vi "Move to Previous Positions.vi"(8 "error in (no error)":errorcluster) -> (0 "error out":errorcluster, 3 "Position Array":dbl[](array[numeric]))   [LabVIEW 2019, in "ESP301.lvlib"]
uses:
  ESP301.lvlib
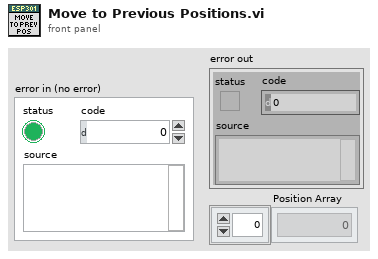
[diagram p1: front panel]
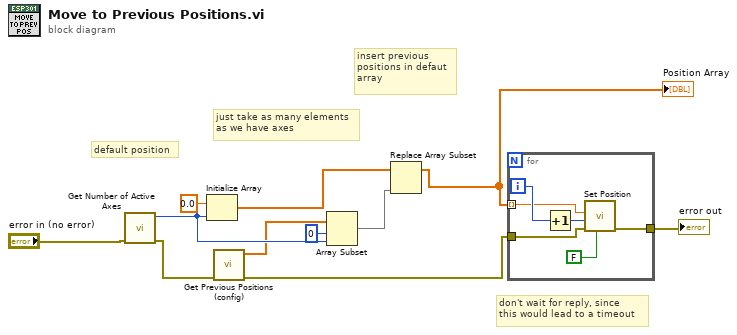
[diagram p0: block diagram]
diagram:
  # "default position"
  # "insert previous\npositions in defaut\narray"
  # "just take as many elements\nas we have axes"
  # "don't wait for reply, since\nthis would lead to a timeout"
  n1 = call "Get Number of Active Axes.vi"("error in (no error)"="error in (no error)") -> ("error out"=w9:errorcluster, "value"=w6:i32)  [unwired: 9 in]
  n2 = Initialize Array(0.0 ("element"), w6) -> (w3:dbl[])
  n3 = call "Get Previous Positions (config).vi"("error in (no error)"=w9) -> ("error out"=w10:errorcluster, "Previous Positions"=w4:dbl[])  [unwired: 9 in]
  n4 = Array Subset(array=w4, index=0, length=w6) -> (w2:dbl[])
  n5 = Replace Array Subset(array=w3, new element=w2) -> (w1:dbl[])  [unwired: 1 in]
  "Position Array" <- w1
  n6 = for {
    tunnel: w1 -> [w14] mode=indexing
    tunnel: w10 -> [w13]
    tunnel: [w12] -> w7
    i -> [w16]
    n7 = Increment(x=w16) -> (x+1=w15:i32)
    n8 = call "Set Position.vi"("wait for reply (T)"=FALSE, "error in (no error)"=w13, "Axis"=w15, "Position"=w14) -> ("error out"=w12:errorcluster)  [unwired: 5 in, 2 out]
  }
  "error out" <- w7
